vi "Generate Header or Footer String.vi"(4 "Right Text":string, 6 "Center Text":string, 7 "Font Tag":string, 8 "error in (no error)":errorcluster, 9 "Left Text":string, 10 "size":enum16{"H1", "H2", "H3", "H4", "H5", "H6", "H7"}(ring), 11 "HTML in":string) -> (0 "error out":errorcluster, 3 "HTML out":string)   [LabVIEW 2017, in "NI_ReportGenerationCore.lvlib"]
uses:
  <vilib>/Utility/NIReport.llb/NI_ReportGenerationCore.lvlib
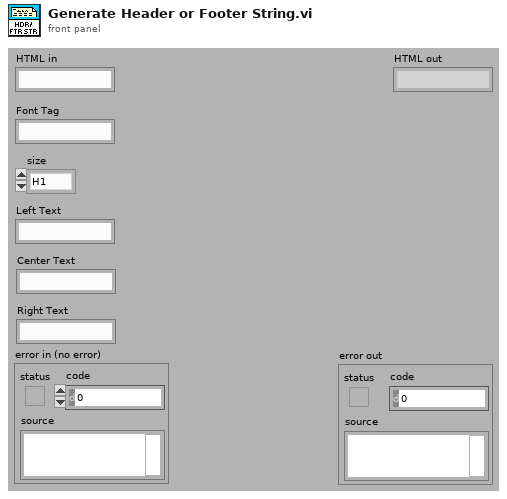
[diagram p1: front panel]
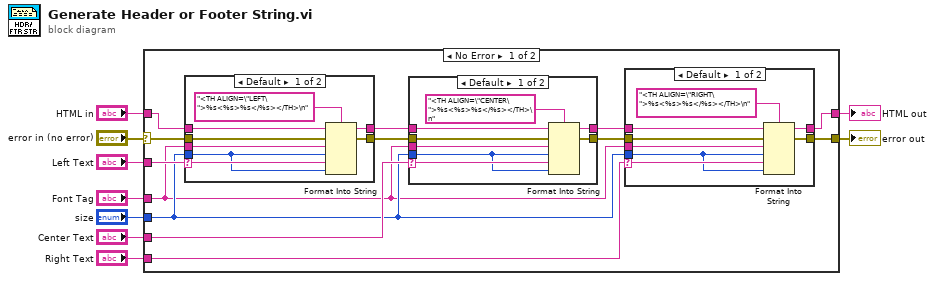
[diagram p0: block diagram]
diagram:
  n1 = case shown="No Error" "error in (no error)" {
    selector: "error in (no error)" -> [w12 w54]
    tunnel: "Font Tag" -> [w10 _]
    tunnel: [w22 w54] -> w8
    tunnel: "Right Text" -> [w21 _]
    tunnel: "Center Text" -> [w20 _]
    tunnel: "Left Text" -> [w19 _]
    tunnel: "HTML in" -> [w18 w53]
    tunnel: [w17 w53] -> w3
    tunnel: "size" -> [w11 _]
    frame No Error {
      n2 = case shown="Default" w19 {
        selector: w19 -> [w45 _]
        tunnel: [w49 w51] -> w13
        tunnel: [w48 w52] -> w14
        tunnel: w12 -> [w50 w52]
        tunnel: w11 -> [w44 _]
        tunnel: w18 -> [w46 w51]
        tunnel: w10 -> [w43 _]
        frame Default {
          n3 = Format Into String(format string="<TH ALIGN=\"LEFT\">%s<%s>%s</%s></TH>\n" ("Format String"), initial string=w46, error in=w50, w43, w44, w45, w44) -> (resulting string=w49:string, error out=w48:errorcluster)
        }
        frame "" {
        }
      }
      n4 = case shown="Default" w20 {
        selector: w20 -> [w35 _]
        tunnel: [w38 w41] -> w15
        tunnel: [w37 w42] -> w16
        tunnel: w14 -> [w40 w42]
        tunnel: w13 -> [w39 w41]
        tunnel: w11 -> [w34 _]
        tunnel: w10 -> [w33 _]
        frame Default {
          n5 = Format Into String(format string="<TH ALIGN=\"CENTER\">%s<%s>%s</%s></TH>\n" ("Format String"), initial string=w39, error in=w40, w33, w34, w35, w34) -> (resulting string=w38:string, error out=w37:errorcluster)
        }
        frame "" {
        }
      }
      n6 = case shown="Default" w21 {
        selector: w21 -> [w25 _]
        tunnel: [w29 w31] -> w17
        tunnel: [w28 w32] -> w22
        tunnel: w16 -> [w27 w32]
        tunnel: w15 -> [w30 w31]
        tunnel: w11 -> [w24 _]
        tunnel: w10 -> [w23 _]
        frame Default {
          n7 = Format Into String(format string="<TH ALIGN=\"RIGHT\">%s<%s>%s</%s></TH>\n" ("Format String"), initial string=w30, error in=w27, w23, w24, w25, w24) -> (resulting string=w29:string, error out=w28:errorcluster)
        }
        frame "True" {
        }
      }
    }
    frame Error {
    }
  }
  "error out" <- w8
  "HTML out" <- w3
